vi "SwerveDrivePoseEst2_InterpRecord_New.vi"(9 "ModulePositions":T1[](array[typedef]) {"Angle"."SIN" format="%13.4f"; "Angle"."COS" format="%13.4f"; "Angle"."VALUE" format="%13.4f"}, 10 "GyroAngle":T2 {"SIN" format="%13.4f"; "COS" format="%13.4f"; "VALUE" format="%13.4f"}, 11 "M_POSE_Meters":T3 {"ROTATION"."SIN" format="%13.4f"; "ROTATION"."COS" format="%13.4f"; "ROTATION"."VALUE" format="%13.4f"; "TRANSLATION"."Y" format="%14.3f"; "TRANSLATION"."X" format="%14.3f"}) -> (3 "SWERVE_DRIVE_POSE_EST2_INTERP_RECORD":T5 {"ModulePositions"."Angle"."SIN" format="%13.4f"; "ModulePositions"."Angle"."COS" format="%13.4f"; "ModulePositions"."Angle"."VALUE" format="%13.4f"; "GyroAngle"."SIN" format="%13.4f"; "GyroAngle"."COS" format="%13.4f"; "GyroAngle"."VALUE" format="%13.4f"; "PoseMeters"."ROTATION"."SIN" format="%13.4f"; "PoseMeters"."ROTATION"."COS" format="%13.4f"; "PoseMeters"."ROTATION"."VALUE" format="%13.4f"; "PoseMeters"."TRANSLATION"."Y" format="%14.3f"; "PoseMeters"."TRANSLATION"."X" format="%14.3f"})   [LabVIEW 2019, in "Trajectory_Library.lvlib"]
doc: "Create a new SwerveDrivePoseEstimator2 Interpolation record.\n\nThis is an internal routine. It should NOT be used by the end user."
uses:
  Trajectory_Library.lvlib
  TypeDef/ROTATION2D.ctl
  TypeDef/TRANSLATION2D.ctl
  TypeDef/POSE2D.ctl
  TypeDef/SWERVE_DRIVE_MODULE_POSITION.ctl
  TypeDef/SWERVE_DRIVE_POSE_EST2_INTERP_RECORD.ctl
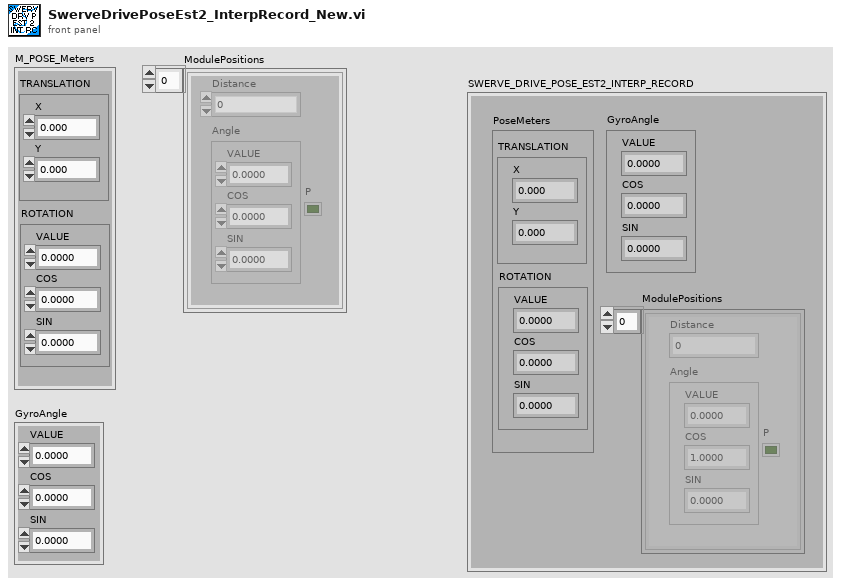
[diagram p1: front panel]
types:
  T1 = typedef "Trajectory_Library.lvlib/SWERVE_DRIVE_MODULE_POSITION.ctl" = cluster{"Distance":dbl, "Angle":T2, "P":bool}
  T2 = typedef "Trajectory_Library.lvlib/ROTATION2D.ctl" = cluster{"VALUE":dbl, "COS":dbl, "SIN":dbl}
  T3 = typedef "Trajectory_Library.lvlib/POSE2D.ctl" = cluster{"TRANSLATION":T4, "ROTATION":T2}
  T4 = typedef "Trajectory_Library.lvlib/TRANSLATION2D.ctl" = cluster{"X":dbl, "Y":dbl}
  T5 = typedef "Trajectory_Library.lvlib/SWERVE_DRIVE_POSE_EST2_INTERP_RECORD.ctl" = cluster{"PoseMeters":T3, "GyroAngle":T2, "ModulePositions":T1[]}
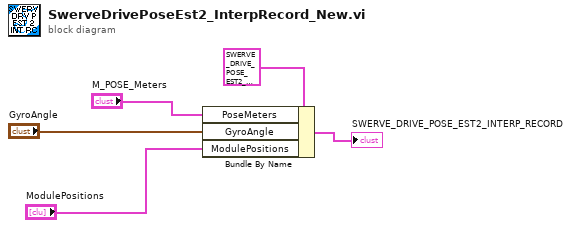
[diagram p0: block diagram]
diagram:
  n1 = Bundle By Name(cluster=T5 {"PoseMeters"={"TRANSLATION"={"X"=0.0, "Y"=0.0}, "ROTATION"={"VALUE"=0.0, "COS"=1.0, "SIN"=0.0}}, "GyroAngle"={"VALUE"=0.0, "COS"=1.0, "SIN"=0.0}, "ModulePositions"=[]} ("SWERVE_DRIVE_POSE_EST2_INTERP_RECORD"), "PoseMeters"="M_POSE_Meters", "GyroAngle"="GyroAngle", "ModulePositions"="ModulePositions") -> (→"SWERVE_DRIVE_POSE_EST2_INTERP_RECORD":T5)
